vi "Thev-Compute Response.vi"(0 "Mag":dbl[][](array[numeric]), 1 "Stimulus":dbl[](array[numeric]), 5 "Phase":dbl[][](array[numeric]), 7 "df (Hz)":dbl, 9 "Probe Mic Gain (dB)":dbl=50000.0, 11 "error in (no error)":errorcluster, 12 "Attenuation (dB)":dbl) -> (4 "ASTF Mag":dbl[](array[numeric]), 6 "ASTF Phase":dbl[](array[numeric]), 8 "Frequency":dbl[](array[numeric]), 15 "error out":errorcluster)   [LabVIEW 2015]
uses:
  Utility VIs/Math VIs/LinSpace (x0-dx-npts).vi
  Utility VIs/Math VIs/FFT x(t) to dB,Degrees (1D).vi
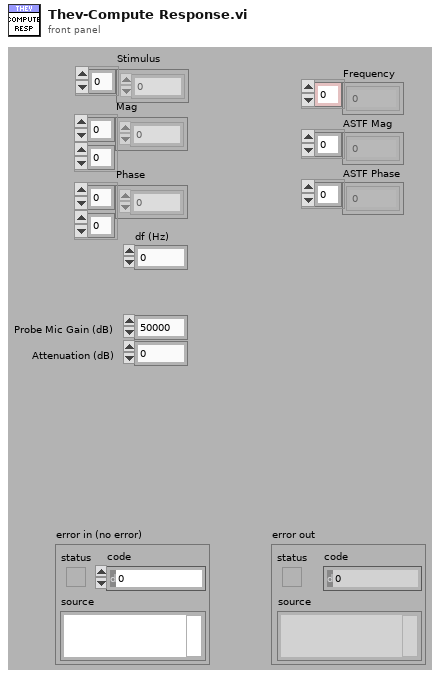
[diagram p1: front panel]
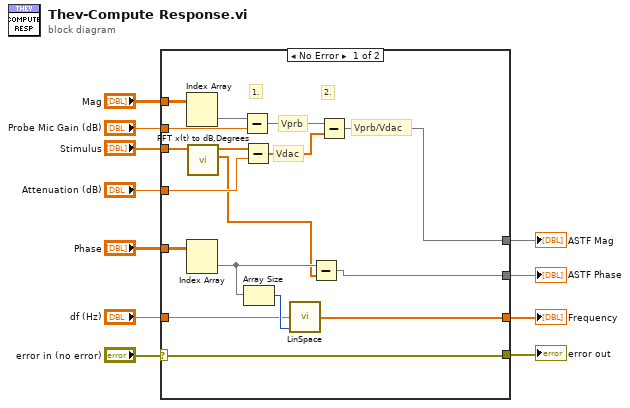
[diagram p0: block diagram]
diagram:
  n1 = case shown="No Error" "error in (no error)" {
    selector: "error in (no error)" -> [w12 w29]
    tunnel: "Mag" -> [w28 _]
    tunnel: "Phase" -> [w27 _]
    tunnel: [w15 _] -> w1
    tunnel: [w14 _] -> w9
    tunnel: "Stimulus" -> [w20 _]
    tunnel: "df (Hz)" -> [w17 _]
    tunnel: [w13 _] -> w5
    tunnel: "Probe Mic Gain (dB)" -> [w23 _]
    tunnel: [w12 w29] -> w3
    tunnel: "Attenuation (dB)" -> [w21 _]
    frame No Error {
      # "2."
      # "1."
      # "Vprb/Vdac"
      # "Vdac"
      # "Vprb"
      n2 = Index Array(array=w28) -> (element=w22:dbl[])  [unwired: 2 in]
      n3 = Index Array(array=w27) -> (element=w26:dbl[])  [unwired: 2 in]
      n4 = call-poly "FFT x(t) to dB,Degrees.vi"("X"=w20) -> ("+Freq Phase of FFT (degrees)"=w16:dbl[], "+Freq. Mag of FFT (dB rms)"=w18:dbl[])  [unwired: 8 in, 1 out]
      n5 = Subtract(x=w22, y=w23) -> (x-y=w24:dbl[])
      n6 = Subtract(x=w18, y=w21) -> (x-y=w19:dbl[])
      n7 = Array Size(array=w26) -> (size(s)=w25:i32)
      n8 = call-poly "LinSpace.vi"("npts"=w25, "dx"=w17) -> ("Array"=w13:dbl[])  [unwired: 2 in, 1 out]
      n9 = Subtract(x=w26, y=w16) -> (x-y=w14:dbl[])
      n10 = Subtract(x=w24, y=w19) -> (x-y=w15:dbl[])
    }
    frame Error {
    }
  }
  "ASTF Mag" <- w1
  "ASTF Phase" <- w9
  "error out" <- w3
  "Frequency" <- w5
